vi "Periodic Tasks.vi"(7 "Chassis X SPD":dbl=0.65, 8 "error in":errorcluster) -> ()   [LabVIEW 2019]
doc: "This VI runs in parallel to other tasks. It can contain as many user-defined periodic loops as you need. These can carry out PID or other sorts of timed response."
uses:
  Robot Global Data.vi
  <vilib>/Rock Robotics/Network Tables/NT Write Number.vi
  <vilib>/Rock Robotics/Network Tables/NT Read Number.vi
  <vilib>/Rock Robotics/WPI/RobotDrive/WPI_RobotDriveArcadeDrive_Standard(NoSaturation).vi
  <vilib>/Rock Robotics/WPI/ThirdParty/REV Robotics/SPARK MAX/Typedef/Spark MAX Control Type.ctl
  <vilib>/Rock Robotics/Network Tables/NT Read Boolean.vi
panel:
  in  "h1":dbl
  in  "a1":dbl
  in  "Chassis Y SPD":dbl=0.65
  # "The tilt applied to the Limelight when mounted"
  # "Height of the floor to the center of the limelight"
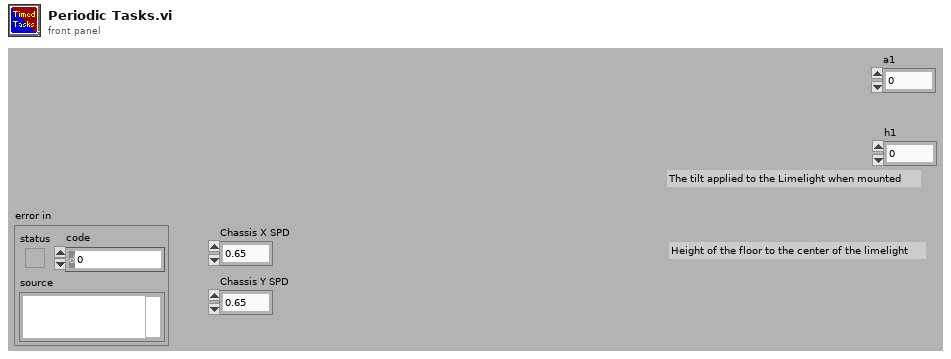
[diagram p1: front panel]
types:
  T1 = typedef "WPI_JoystickDevRef.ctl" = cluster{"Device":T2}
  T2 = typedef "WPI_JoystickDeviceEnum.ctl" = enum16{"USB 0", "USB 1", "USB 2", "USB 3", "USB 4", "USB 5"}
  T3 = typedef "WPI_RobotDriveDevRef.ctl" = cluster{"DevStatus":errorcluster, "Motors[]":T4[], "Square Inputs":bool, "Max Output":dbl}
  T4 = typedef "WPI_MotorControlDeviceRef.ctl" = cluster{"DeviceStatus":errorcluster, "Type":T5, "PWM":cluster{"PWM Channel":T6, "DeadBand":T7}, "CAN":cluster{"Device Number":u8, "SetOutput VI Ref":variant, "GetOutput VI Ref":variant, "Enable VI Ref":variant, "Disable VI Ref":variant, "Data":variant}, "Invert":bool, "DIO PWM":cluster{"PWM \"Enable\" Channel":T6, "DIOChannel":T8, "PWM Rate":dbl}}
  T5 = typedef "WPI_MotorControlType.ctl" = enum16{"PWM", "CAN", "DIO PWM"}
  T6 = typedef "FPGA_DIOPWMChannel.ctl" = enum8{"PWM 0", "PWM 1", "PWM 2", "PWM 3", "PWM 4", "PWM 5", "PWM 6", "PWM 7", "PWM 8", "PWM 9", "PWM MXP 0", "PWM MXP 1", "PWM MXP 2", "PWM MXP 3", "PWM MXP 4", "PWM MXP 5", "PWM MXP 6", "PWM MXP 7", "PWM MXP 8", "PWM MXP 9", "Invalid"}
  T7 = typedef "WPI_PWMDeadband.ctl" = cluster{"Name":string, "maxPositivePwm":i32, "minPositivePwm":i32, "centerPwm":i32, "maxNegativePwm":i32, "minNegativePwm":i32, "angularRange":u16}
  T8 = typedef "FPGA_DIOChannel.ctl" = enum8{"DIO 0", "DIO 1", "DIO 2", "DIO 3", "DIO 4", "DIO 5", "DIO 6", "DIO 7", "DIO 8", "DIO 9", "DIO MXP 0", "DIO MXP 1", "DIO MXP 2", "DIO MXP 3", "DIO MXP 4", "DIO MXP 5", "DIO MXP 6", "DIO MXP 7", "DIO MXP 8", "DIO MXP 9", "DIO MXP 10", "DIO MXP 11", "DIO MXP 12", "DIO MXP 13", "DIO MXP 14", "DIO MXP 15", "SPI Port CS1", "SPI Port CS2", "SPI Port CS3", "SPI Port MISO", "SPI Port MOSI", "Invalid"}
  T9 = cluster{"JoystickDevRef":T1, "RobotDriveDevRef":T3}
  T10 = typedef "Spark MAX Control Type.ctl" = enum16{"Percent VBus", "Voltage", "Velocity", "Position", "Smart Motion", "Current", "Smart Velocity"}
  T11 = typedef "WPI_ServoDeviceRef.ctl" = cluster{"DeviceStatus":errorcluster, "PWM Channel":T6, "DeadBand":T7}
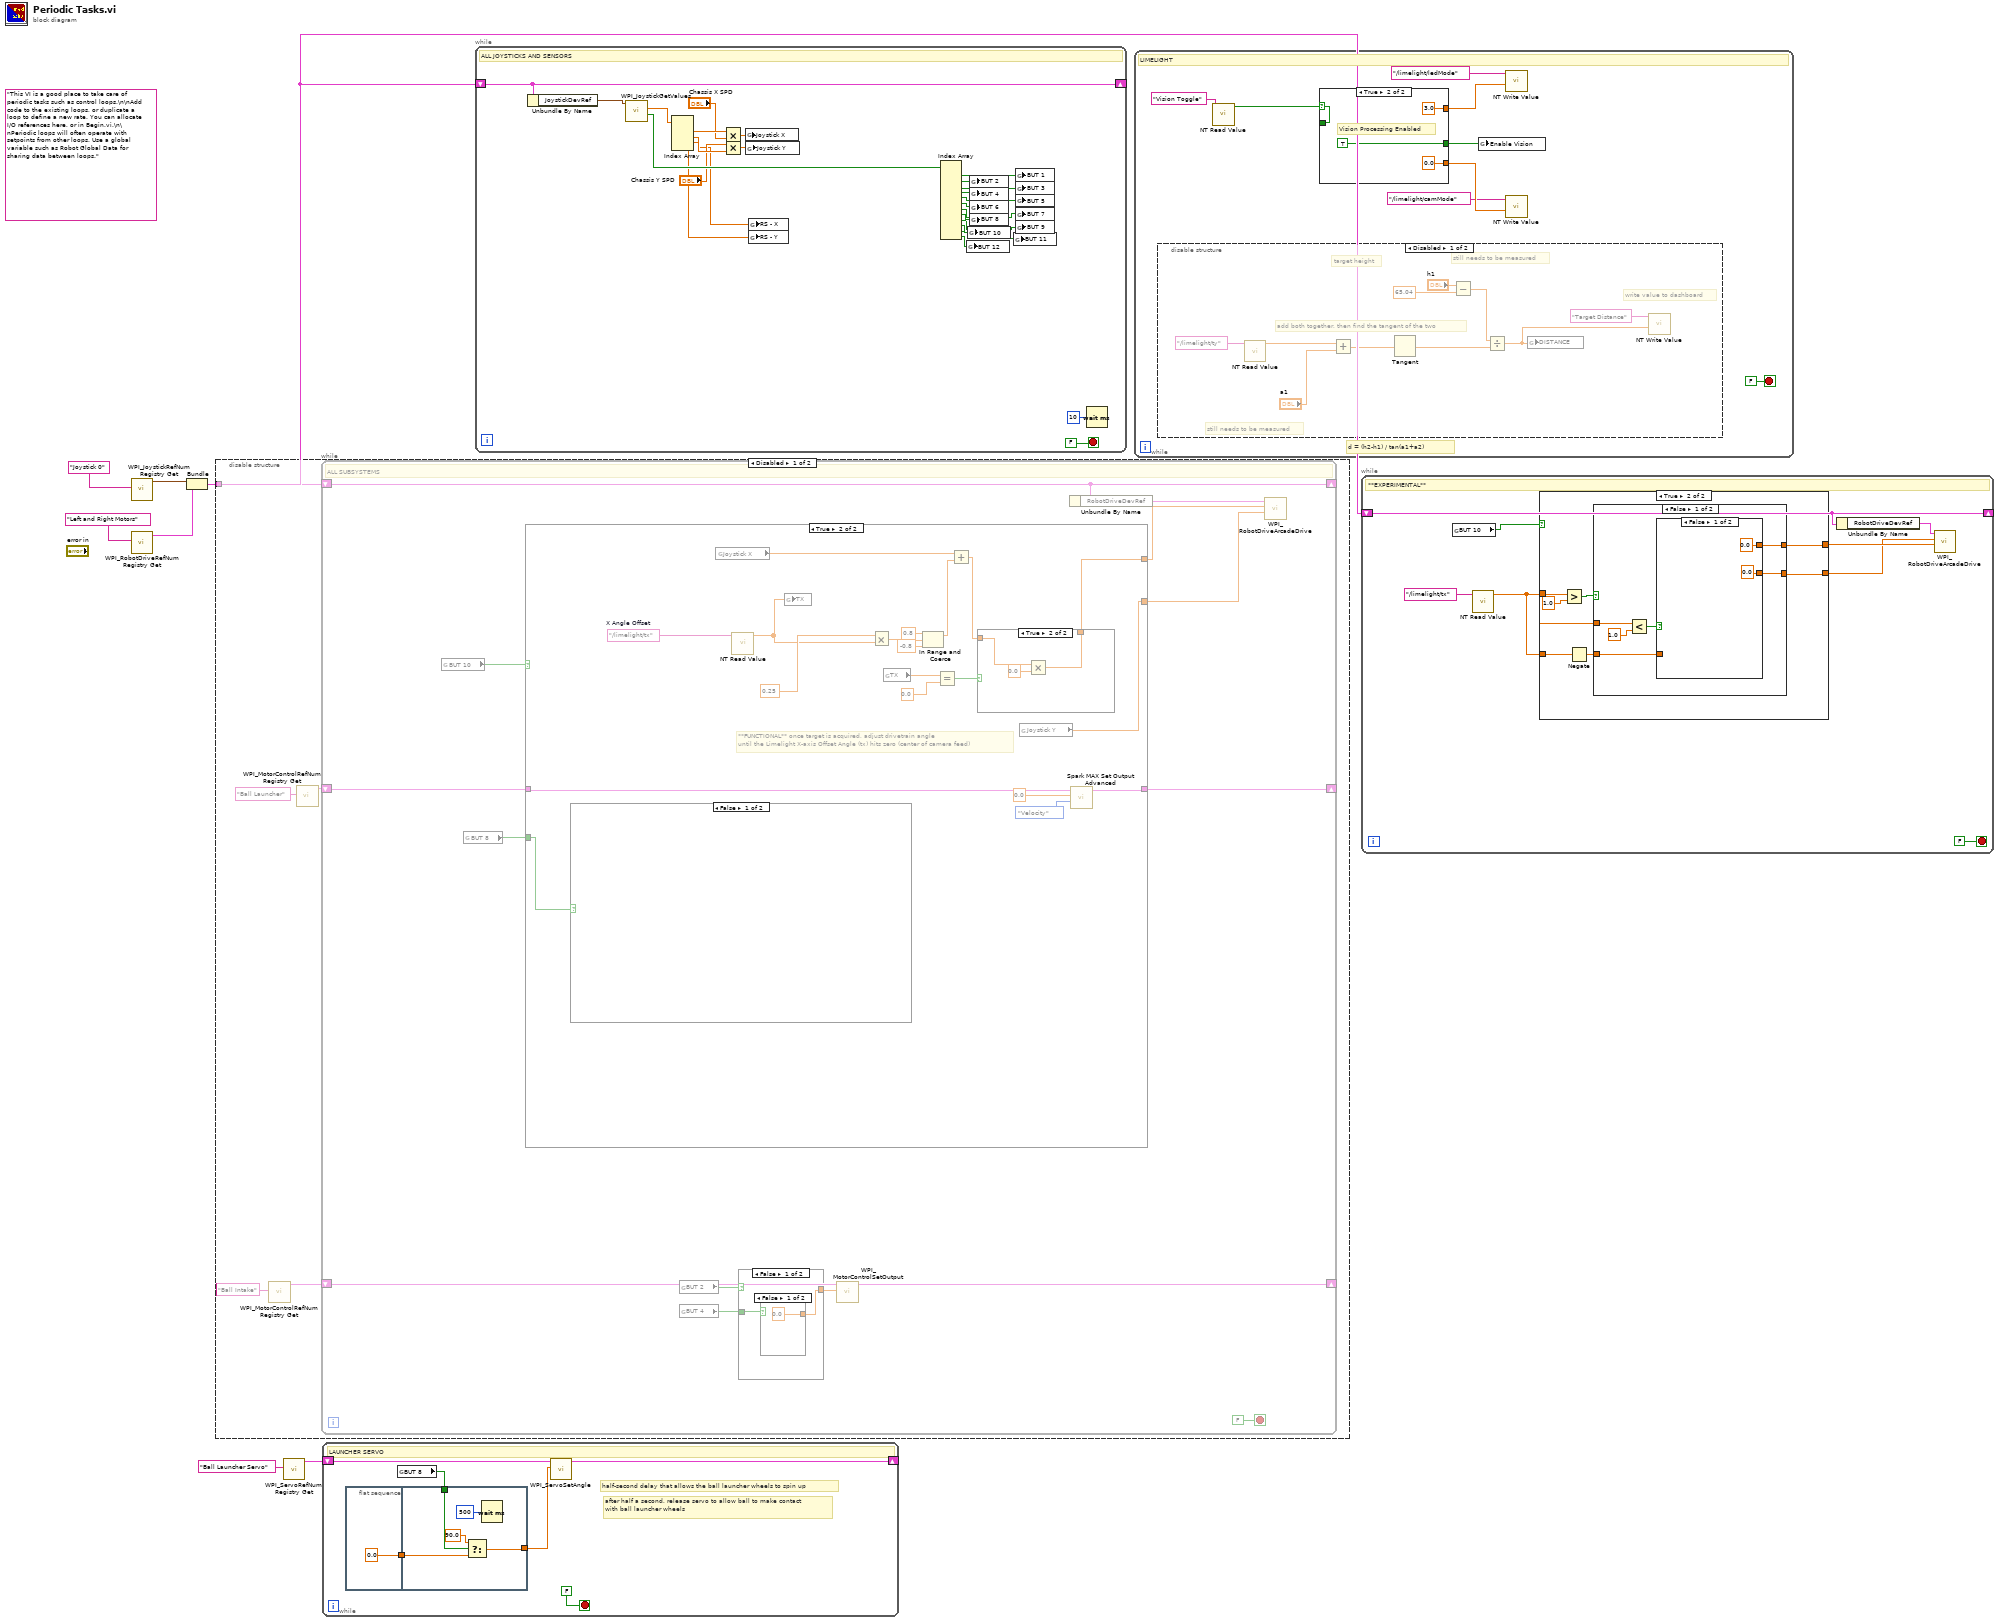
[diagram p0: block diagram]
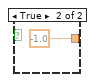
[diagram p2: hidden frame]
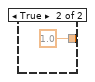
[diagram p3: hidden frame]
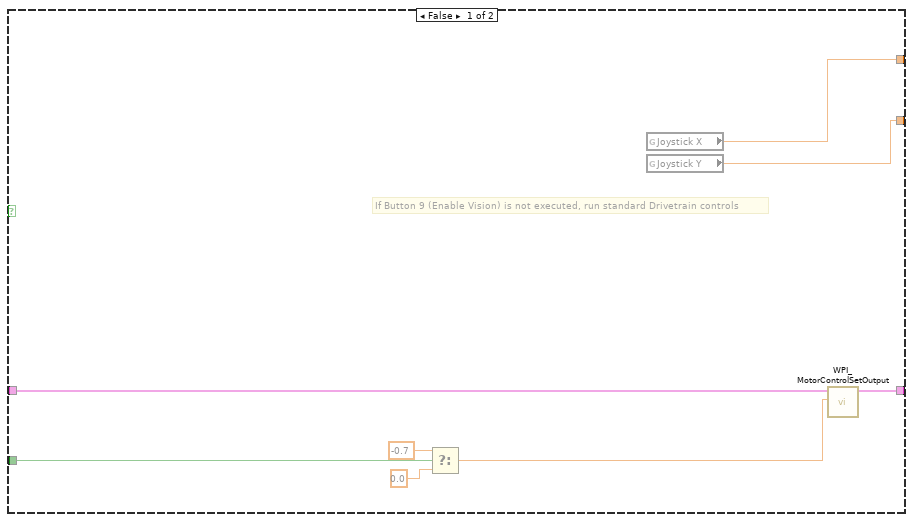
[diagram p4: hidden frame]
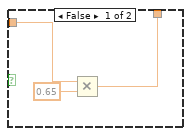
[diagram p6: hidden frame]
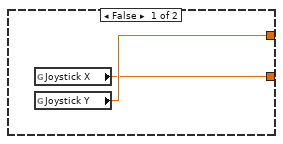
[diagram p8: hidden frame]
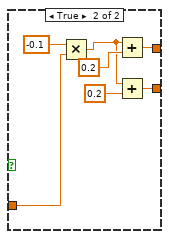
[diagram p9: hidden frame]
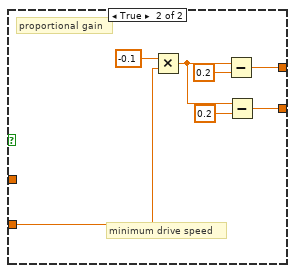
[diagram p10: hidden frame]
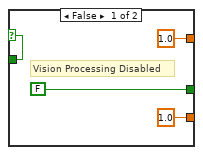
[diagram p12: hidden frame]
diagram:
  (unwired) "This VI is a good place to take care of periodic tasks such as control loops.\n\nAdd code to the existing loops, or duplicate a loop to define a new rate. You can allocate I/O references here, or in Begin.vi.\n\nPeriodic loops will often operate with setpoints from other loops. Use a global variable such as Robot Global Data for sharing data between loops."
  n1 = call <vilib>:"WPI_JoystickRefNum Registry Get.vi"("refnum name"="Joystick 0") -> ("JoystickDevRef"=w5:T1)  [unwired: 1 in, 9 out]
  n2 = call <vilib>:"WPI_RobotDriveRefNum Registry Get.vi"("refnum name"="Left and Right Motors") -> ("RobotDriveDevRef"=w4:T3)  [unwired: 1 in, 9 out]
  n3 = Bundle("JoystickDevRef"=w5, "RobotDriveDevRef"=w4) -> (w1:T9)  [unwired: 1 out]
  n4 = disable-structure shown="Disabled" {
    disable-tunnel: w1 -> [w8 _]
    frame Disabled {
      n5 = call <vilib>:"WPI_MotorControlRefNum Registry Get.vi"("refnum name"="Ball Intake") -> ("MotorControlDevRef"=w10:T4)  [unwired: 9 in, 1 out]
      n6 = call <vilib>:"WPI_MotorControlRefNum Registry Get.vi"("refnum name"="Ball Launcher") -> ("MotorControlDevRef"=w12:T4)  [unwired: 9 in, 1 out]
      n7 = while {
        shift-right: [w25] -> _
        shift-left: w8 -> [w25]
        shift-right: [w18] -> _
        shift-left: w12 -> [w19]
        shift-right: [w14] -> _
        shift-left: w10 -> [w13]
        stop <- FALSE stop-if-true
        # "ALL SUBSYSTEMS"
        n8 = global read "Robot Global Data.vi" "BUT 10"() -> (w24:bool)
        n9 = global read "Robot Global Data.vi" "BUT 8"() -> (w20:bool)
        n10 = case shown="True" w24 {
          tunnel: [w39 w49] -> w22
          tunnel: [w38 w45] -> w21
          tunnel: w20 -> [w33 w44]
          tunnel: w19 -> [w36 w42]
          tunnel: [w37 w43] -> w18
          frame False {
            # "If Button 9 (Enable Vision) is not executed, run standard Drivetrain controls"
            n11 = Select(t=-0.7, s=w33, f=0.0) -> (s? t:f=w35:dbl)
            n12 = global read "Robot Global Data.vi" "Joystick X"() -> (w39:dbl)
            n13 = global read "Robot Global Data.vi" "Joystick Y"() -> (w38:dbl)
            n14 = call <vilib>:"WPI_MotorControlSetOutput.vi"("Output"=w35, "MotorControlDevRef"=w36) -> ("MotorControlDevRef"=w37:T4)  [unwired: 7 in, 2 out]
          }
          frame True {
            w58 = "/limelight/tx"  # X Angle Offset
            # "**FUNCTIONAL** once target is acquired, adjust drivetrain angle \nuntil the Limelight X-axis Offset Angle (tx) hits zero (center of camera feed)"
            n15 = case shown="False" w44 {
              frame False {
              }
              frame True {
              }
            }
            n16 = global read "Robot Global Data.vi" "Joystick X"() -> (w57:dbl)
            n17 = call-poly <vilib>:"NT Read Value.vi"("Name"=w58) -> ("Numeric"=w51:dbl)  [unwired: 9 in, 1 out]
            n18 = global write "Robot Global Data.vi" "TX"(w51) -> ()
            n19 = Multiply(x=0.25 ("y"), y=w51) -> (x*y=w55:dbl)
            n20 = global read "Robot Global Data.vi" "TX"() -> (w47:dbl)
            n21 = In Range and Coerce(upper limit=0.8, x=w55, lower limit=-0.8) -> (coerced(x)=w56:dbl)  [unwired: 1 out]
            n22 = Equal?(x=w47, y=0.0) -> (x = y?=w48:bool)
            n23 = Add(x=w57, y=w56) -> (x+y=w50:dbl)
            n24 = case shown="True" w48 {
              tunnel: w50 -> [w60 w64]
              tunnel: [w61 w62] -> w49
              frame False {
                n25 = Multiply(x=w60, y=0.65) -> (x*y=w61:dbl)
              }
              frame True {
                n26 = Multiply(x=w64, y=0.0) -> (x*y=w62:dbl)
              }
            }
            n27 = global read "Robot Global Data.vi" "Joystick Y"() -> (w45:dbl)
            n28 = call <vilib>:"Spark MAX Set Output Advanced.vi"("Control Mode"=Spark_MAX_Control_Type."Velocity", "Setpoint"=0.0, "MotorControlDevRef"=w42) -> ("MotorControlDevRef"=w43:T4)  [unwired: 7 in, 1 out]
          }
        }
        n29 = global read "Robot Global Data.vi" "BUT 2"() -> (w16:bool)
        n30 = global read "Robot Global Data.vi" "BUT 4"() -> (w17:bool)
        n31 = case shown="False" w16 {
          tunnel: [w28 1.0 ("Output")] -> w15
          tunnel: w17 -> [w27 _]
          frame False {
            n32 = case shown="False" w27 {
              tunnel: [0.0 ("Output") -1.0 ("Output")] -> w28
              frame False {
              }
              frame True {
              }
            }
          }
          frame True {
          }
        }
        n33 = call <vilib>:"WPI_MotorControlSetOutput.vi"("Output"=w15, "MotorControlDevRef"=w13) -> ("MotorControlDevRef"=w14:T4)  [unwired: 7 in, 2 out]
        n34 = Unbundle By Name(w25) -> ("RobotDriveDevRef"=w23:T3)
        n35 = call-poly <vilib>:"WPI_RobotDriveArcadeDrive.vi"("Y axis value"=w21, "X axis value"=w22, "RobotDriveDevRef"=w23) -> ()  [unwired: 6 in, 3 out]
      }
    }
    frame Enabled {
    }
  }
  n36 = call <vilib>:"WPI_ServoRefNum Registry Get.vi"("refnum name"="Ball Launcher Servo") -> ("ServoDeviceRef"=w3:T11)  [unwired: 9 in, 1 out]
  n37 = while {
    shift-right: [w66] -> _
    shift-left: w3 -> [w67]
    stop <- FALSE stop-if-true
    # "after half a second, release servo to allow ball to make contact\nwith ball launcher wheels"
    # "half-second delay that allows the ball launcher wheels to spin up"
    # "LAUNCHER SERVO"
    n38 = flat-sequence {
      tunnel: [0.0 ("f")] -> w70
      tunnel: [w75] -> w69
      tunnel: w68 -> [w74]
      tunnel: w70 -> [w72]
      frame #0 {
      }
      frame #1 {
        n39 = Select(t=90.0, s=w74, f=w72) -> (s? t:f=w75:dbl)
        n40 = Wait (ms)(milliseconds to wait=u32 500) -> ()  [unwired: 1 out]
      }
    }
    n41 = global read "Robot Global Data.vi" "BUT 8"() -> (w68:bool)
    n42 = call <vilib>:"WPI_ServoSetAngle.vi"("Angle"=w69, "ServoDeviceRef"=w67) -> ("ServoDeviceRef"=w66:T11)  [unwired: 8 in, 1 out]
  }
  n43 = while {
    shift-right: [w86] -> _
    shift-left: w1 -> [w86]
    stop <- FALSE stop-if-true
    # "ALL JOYSTICKS AND SENSORS"
    n44 = Unbundle By Name(w86) -> ("JoystickDevRef"=w100:T1)
    n45 = call <vilib>:"WPI_JoystickGetValues.vi"("JoystickDevRef"=w100) -> ("Buttons"=w99:bool[], "Axes"=w85:dbl[])  [unwired: 6 in, 3 out]
    n46 = Index Array(array=w85) -> (element #1=w82:dbl, element #2=w81:dbl, element #3=w78:dbl, element #4=w77:dbl)  [unwired: 4 in]
    n47 = Multiply(x=w82, y="Chassis X SPD") -> (x*y=w84:dbl)
    n48 = Multiply(x="Chassis Y SPD", y=w81) -> (x*y=w83:dbl)
    n49 = global write "Robot Global Data.vi" "Joystick X"(w84) -> ()
    n50 = global write "Robot Global Data.vi" "Joystick Y"(w83) -> ()
    n51 = global write "Robot Global Data.vi" "RS - X"(w78) -> ()
    n52 = global write "Robot Global Data.vi" "RS - Y"(w77) -> ()
    n53 = Index Array(array=w99) -> (element #1=w98:bool, element #2=w97:bool, element #3=w96:bool, element #4=w95:bool, element #5=w94:bool, element #6=w93:bool, element #7=w92:bool, element #8=w91:bool, element #9=w90:bool, element #10=w89:bool, element #11=w88:bool, element #12=w87:bool)  [unwired: 12 in]
    n54 = global write "Robot Global Data.vi" "BUT 12"(w87) -> ()
    n55 = global write "Robot Global Data.vi" "BUT 10"(w89) -> ()
    n56 = global write "Robot Global Data.vi" "BUT 2"(w97) -> ()
    n57 = global write "Robot Global Data.vi" "BUT 4"(w95) -> ()
    n58 = global write "Robot Global Data.vi" "BUT 6"(w93) -> ()
    n59 = global write "Robot Global Data.vi" "BUT 8"(w91) -> ()
    n60 = global write "Robot Global Data.vi" "BUT 11"(w88) -> ()
    n61 = global write "Robot Global Data.vi" "BUT 1"(w98) -> ()
    n62 = global write "Robot Global Data.vi" "BUT 3"(w96) -> ()
    n63 = global write "Robot Global Data.vi" "BUT 5"(w94) -> ()
    n64 = global write "Robot Global Data.vi" "BUT 7"(w92) -> ()
    n65 = global write "Robot Global Data.vi" "BUT 9"(w90) -> ()
    n66 = Wait (ms)(milliseconds to wait=u32 10) -> ()  [unwired: 1 out]
  }
  n67 = while {
    stop <- FALSE stop-if-true
    # "d = (h2-h1) / tan(a1+a2)"
    # "LIMELIGHT"
    n68 = disable-structure shown="Disabled" {
      frame Disabled {
        # "write value to dashboard"
        # "still needs to be measured"
        # "target height"
        # "add both together, then find the tangent of the two"
        # "still needs to be measured"
        n69 = call-poly <vilib>:"NT Read Value.vi"("Name"="/limelight/ty") -> ("Numeric"=w119:dbl)  [unwired: 9 in, 1 out]
        n70 = Add(x=w119, y="a1") -> (x+y=w117:dbl)
        n71 = Tangent(1:w117) -> (0:w116:dbl)
        n72 = Subtract(x="h1", y=65.04) -> (x-y=w114:dbl)
        n73 = Divide(x=w114, y=w116) -> (x/y=w111:dbl)
        n74 = global write "Robot Global Data.vi" "DISTANCE"(w111) -> ()
        n75 = call-poly <vilib>:"NT Write Value.vi"("Numeric"=w111, "Name"="Target Distance") -> ()  [unwired: 9 in, 1 out]
      }
      frame Enabled {
      }
    }
    n76 = call-poly <vilib>:"NT Read Value.vi"("Name"="Vision Toggle") -> ("Boolean"=w104:bool)  [unwired: 9 in, 1 out]
    n77 = case shown="True" w104 {
      selector: w104 -> [w121 w125]
      tunnel: [FALSE ("Enable Vision") TRUE ("Enable Vision")] -> w108
      tunnel: [1.0 ("Numeric") 0.0 ("Numeric")] -> w109
      tunnel: [1.0 ("Numeric") 3.0 ("Numeric")] -> w110
      tunnel: [w121 w125] -> _
      frame False {
        # "Vision Processing Disabled"
      }
      frame True {
        # "Vision Processing Enabled"
      }
    }
    n78 = global write "Robot Global Data.vi" "Enable Vision"(w108) -> ()
    n79 = call-poly <vilib>:"NT Write Value.vi"("Numeric"=w110, "Name"="/limelight/ledMode") -> ()  [unwired: 9 in, 1 out]
    n80 = call-poly <vilib>:"NT Write Value.vi"("Numeric"=w109, "Name"="/limelight/camMode") -> ()  [unwired: 9 in, 1 out]
  }
  n81 = while {
    shift-right: [w133] -> _
    shift-left: w1 -> [w133]
    stop <- FALSE stop-if-true
    # "**EXPERIMENTAL**"
    n82 = global read "Robot Global Data.vi" "BUT 10"() -> (w134:bool)
    n83 = call-poly <vilib>:"NT Read Value.vi"("Name"="/limelight/tx") -> ("Numeric"=w129:dbl)  [unwired: 9 in, 1 out]
    n84 = case shown="True" w134 {
      tunnel: w129 -> [_ w143]
      tunnel: [w138 w142] -> w131
      tunnel: [w137 w141] -> w130
      tunnel: w129 -> [_ w140]
      frame False {
        n85 = global read "Robot Global Data.vi" "Joystick X"() -> (w137:dbl)
        n86 = global read "Robot Global Data.vi" "Joystick Y"() -> (w138:dbl)
      }
      frame True {
        n87 = Greater?(x=w143, y=1.0) -> (0:w145:bool)
        n88 = Negate(x=w140) -> (-x=w139:dbl)
        n89 = case shown="False" w145 {
          tunnel: w143 -> [w150 _]
          tunnel: [w148 w167] -> w142
          tunnel: [w147 w166] -> w141
          tunnel: w139 -> [w146 w161]
          frame False {
            n90 = Less?(x=w150, y=1.0) -> (x < y?=w151:bool)
            n91 = case shown="False" w151 {
              tunnel: [0.0 w160] -> w148
              tunnel: [0.0 w159] -> w147
              tunnel: w146 -> [_ w158]
              frame False {
              }
              frame True {
                n92 = Multiply(x=-0.1, y=w158) -> (x*y=w155:dbl)
                n93 = Add(x=w155, y=0.2) -> (x+y=w160:dbl)
                n94 = Add(x=w155, y=0.2) -> (x+y=w159:dbl)
              }
            }
          }
          frame True {
            # "minimum drive speed"
            # "proportional gain"
            n95 = Multiply(x=-0.1, y=w161) -> (x*y=w164:dbl)
            n96 = Subtract(x=w164, y=0.2) -> (x-y=w167:dbl)
            n97 = Subtract(x=w164, y=0.2) -> (x-y=w166:dbl)
          }
        }
      }
    }
    n98 = Unbundle By Name(w133) -> ("RobotDriveDevRef"=w132:T3)
    n99 = call-poly <vilib>:"WPI_RobotDriveArcadeDrive.vi"("Y axis value"=w131, "X axis value"=w130, "RobotDriveDevRef"=w132) -> ()  [unwired: 6 in, 3 out]
  }
